vi "RFID_Checker.vi"(8 "error in (no error)":errorcluster, 11 "Ref in":T1={"MS SQL Connection"=refnum, "UDL File"=path "", "Time"="", "DCODE"="", "WIP+1"=0, "MC No?"=0, "POKAYOKE?"=FALSE, "Expected Result"="", "Result [Status]"="", "Clock"=0.0, "RFID"="", "WIP Queue"=refnum, "TS Parameter"={"ProfitCenterCode"="", "LineCode"="", "WorkOrderNumber"="", "Model"="", "Model_with_Prefix"="", "VendorCode"="", "SetParameterDateCode"="", "PokaYoke"=0, "Target"=1, "Live_DateCode"="", "CustomerPartNumber"="", "Hand"="", "sBarcode"=FALSE, "FCA"=0, "Ent_Stamp"=timestamp(0 s since 1904-01-01), "STS_CD"=0.0}, "Data_Queue"=[], "RFID Serial No."=""} {"TS Parameter"."FCA" format="%01d"; "TS Parameter"."Target" min=1 max=100000; "TS Parameter"."PokaYoke" min=0 max=1}) -> (0 "error out":errorcluster, 1 "TS_BSC":i32, 2 "Message":picture, 3 "Ref out":T1={"MS SQL Connection"=refnum, "UDL File"=path "", "Time"="", "DCODE"="", "WIP+1"=0, "MC No?"=0, "POKAYOKE?"=FALSE, "Expected Result"="", "Result [Status]"="", "Clock"=0.0, "RFID"="", "WIP Queue"=refnum, "TS Parameter"={"ProfitCenterCode"="", "LineCode"="", "WorkOrderNumber"="", "Model"="", "Model_with_Prefix"="", "VendorCode"="", "SetParameterDateCode"="", "PokaYoke"=0, "Target"=1, "Live_DateCode"="", "CustomerPartNumber"="", "Hand"="", "sBarcode"=FALSE, "FCA"=0, "Ent_Stamp"=timestamp(0 s since 1904-01-01), "STS_CD"=0.0}, "Data_Queue"=[], "RFID Serial No."=""} {"TS Parameter"."FCA" format="%01d"; "TS Parameter"."Target" min=1 max=100000; "TS Parameter"."PokaYoke" min=0 max=1}, 5 "Expected Result":string)   [LabVIEW 2020]
uses:
  Controls/TD SQL.ctl
  <vilib>/addons/database/Connection.llb/Conn ObjectReference.ctl
  Controls/WIP_State.ctl
  Controls/TS_Parameter.ctl
  <vilib>/addons/database/NI_Database_API.lvlib
panel:
  out "Act Count":i32
  out "TS_Message":string
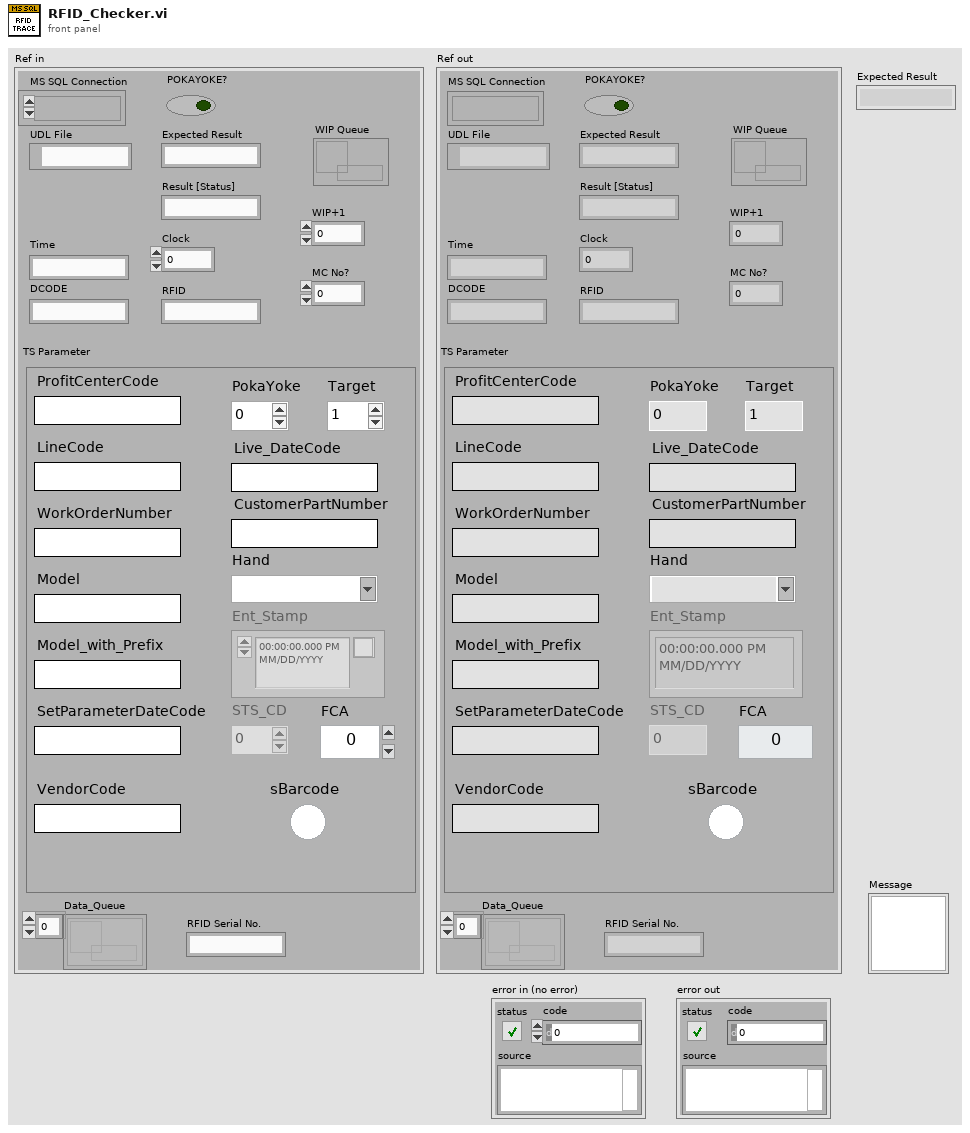
[diagram p1: front panel]
types:
  T1 = typedef "TD SQL.ctl" = cluster{"MS SQL Connection":T2, "UDL File":path, "Time":string, "DCODE":string, "WIP+1":i64, "MC No?":i32, "POKAYOKE?":bool, "Expected Result":string, "Result [Status]":string, "Clock":dbl, "RFID":string, "WIP Queue":refnum<queue>, "TS Parameter":T3, "Data_Queue":refnum<queue>[], "RFID Serial No.":string}
  T2 = typedef "NI_Database_API.lvlib/Conn ObjectReference.ctl" = refnum<k1>
  T3 = typedef "TS_Parameter.ctl" = cluster{"ProfitCenterCode":string, "LineCode":string, "WorkOrderNumber":string, "Model":string, "Model_with_Prefix":string, "VendorCode":string, "SetParameterDateCode":string, "PokaYoke":i32, "Target":i32, "Live_DateCode":string, "CustomerPartNumber":string, "Hand":string, "sBarcode":bool, "FCA":i32, "Ent_Stamp":timestamp, "STS_CD":dbl}
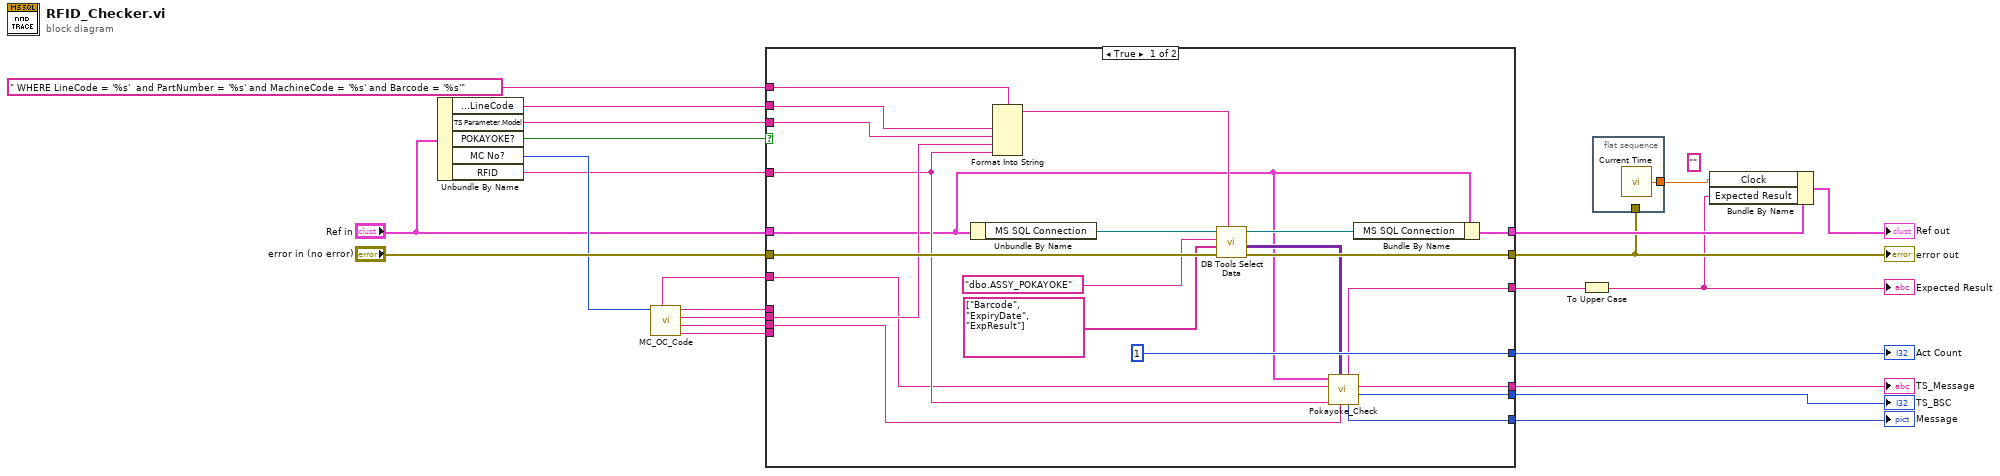
[diagram p0: block diagram]
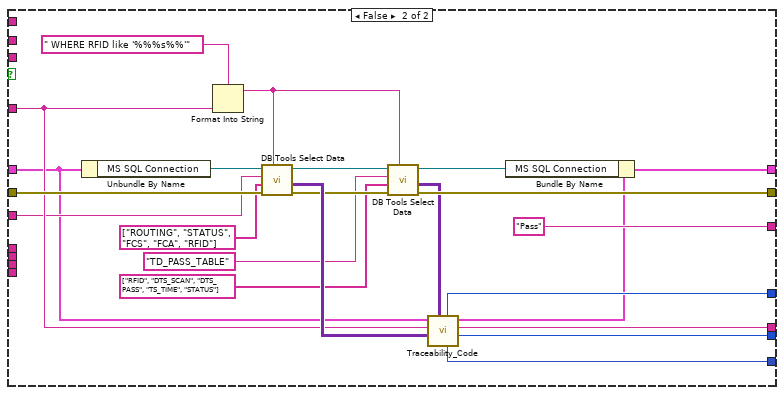
[diagram p2: hidden frame]
diagram:
  (unwired) "" ("RFID")
  n1 = Unbundle By Name("Ref in") -> ("TS Parameter.LineCode"=w1:string, "TS Parameter.Model"=w2:string, "POKAYOKE?"=w10:bool, "MC No?"=w11:i32, "RFID"=w4:string)
  n2 = call "MC_OC_Code.vi"("index"=w11) -> ("Code Query"=w20:string, "TS CODE TAG"=w14:string, "Machine Code"=w21:string, "Operation Code"=w22:string, "Table Name"=w12:string)  [unwired: 4 in, 2 out]
  n3 = case shown="True" w10 {
    tunnel: [w45 w68] -> w15
    tunnel: [w44 w54] -> w5
    tunnel: "error in (no error)" -> [w42 w67]
    tunnel: w4 -> [w35 w63]
    tunnel: [1 ("Act Count") w61] -> w17
    tunnel: [w27 w49] -> w18
    tunnel: [w36 w60] -> w19
    tunnel: "Ref in" -> [w30 w46]
    tunnel: w20 -> [_ _]
    tunnel: w21 -> [w38 _]
    tunnel: w22 -> [_ _]
    tunnel: w12 -> [w29 w59]
    tunnel: [w34 "Pass" ("Expected Result")] -> w7
    tunnel: " WHERE LineCode = '%s'  and PartNumber = '%s' and MachineCode = '%s' and Barcode = '%s'" -> [w33 _]
    tunnel: w14 -> [w26 _]
    tunnel: [w28 w47] -> w13
    tunnel: w2 -> [w25 _]
    tunnel: w1 -> [w24 _]
    frame True {
      n4 = Unbundle By Name(w30) -> ("MS SQL Connection"=w41:T2)
      n5 = Format Into String(format string=w33, w24, w25, w38, w35) -> (resulting string=w40:string)  [unwired: 2 in, 1 out]
      n6 = call <vilib>:"DB Tools Select Data.vi"("condition"=w40, "error in (no error)"=w42, "columns"=string[] ["Barcode", "ExpiryDate", "ExpResult"], "table"="dbo.ASSY_POKAYOKE", "connection reference"=w41) -> ("error out"=w44:errorcluster, "data"=w31:variant[][], "connection reference out"=w43:T2)  [unwired: 1 in]
      n7 = call "Pokayoke_Check.vi"("Tag Name"=w26, "Pokayoke Data"=w31, "RFID"=w35, "Table"=w29, "Ref in"=w30) -> ("TS_BSC"=w27:i32, "TS_Message"=w36:string, "Message"=w28:picture, "Expected Result"=w34:string)  [unwired: 3 in]
      n8 = Bundle By Name(cluster=w30, "MS SQL Connection"=w43) -> (w45:T1)
    }
    frame False {
      n9 = Unbundle By Name(w46) -> ("MS SQL Connection"=w66:T2)
      n10 = Format Into String(format string=" WHERE RFID like '%%%s%%'", w63) -> (resulting string=w53:string)  [unwired: 2 in, 1 out]
      n11 = call <vilib>:"DB Tools Select Data.vi"("condition"=w53, "error in (no error)"=w67, "columns"=string[] ["ROUTING", "STATUS", "FCS", "FCA", "RFID"], "table"=w59, "connection reference"=w66) -> ("error out"=w55:errorcluster, "data"=w64:variant[][], "connection reference out"=w57:T2)  [unwired: 1 in]
      n12 = call <vilib>:"DB Tools Select Data.vi"("condition"=w53, "error in (no error)"=w55, "columns"=string[] ["RFID", "DTS_SCAN", "DTS_PASS", "TS_TIME", "STATUS"], "table"="TD_PASS_TABLE", "connection reference"=w57) -> ("error out"=w54:errorcluster, "data"=w50:variant[][], "connection reference out"=w56:T2)  [unwired: 1 in]
      n13 = call "Traceability_Code.vi"("Return Data [ASR]"=w50, "Return Data"=w64, "RFID"=w63, "Ref in"=w46) -> ("TS_BSC"=w49:i32, "TS_Message"=w60:string, "Ref Out"=w48:T1, "Message"=w47:picture, "Act Count"=w61:i32)  [unwired: 2 in, 1 out]
      n14 = Bundle By Name(cluster=w48, "MS SQL Connection"=w56) -> (w68:T1)
    }
  }
  "TS_Message" <- w19
  "TS_BSC" <- w18
  "Act Count" <- w17
  "error out" <- w5
  "Message" <- w13
  n15 = To Upper Case(1:w7) -> (0:w3:string)
  "Expected Result" <- w3
  n16 = flat-sequence {
    tunnel: [w69] -> w6
    tunnel: w5 -> [_]
    frame #0 {
      n17 = call <userlib>:"Current Time.vi"() -> ("Current Time (Sec)"=w69:dbl)  [unwired: 15 in]
    }
  }
  n18 = Bundle By Name(cluster=w15, "Clock"=w6, "Expected Result"=w3) -> (→"Ref out":T1)
